vi "Remove Unprintable Chars.vi"(1 "input":string caption="Eingang") -> (0 "output":string caption="Ausgang")   [LabVIEW 2009]
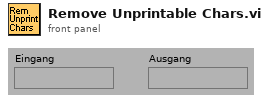
[diagram p1: front panel]
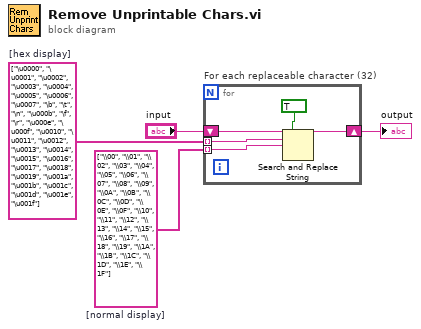
[diagram p0: block diagram]
diagram:
  w2 = string[] ["\u0000", "\u0001", "\u0002", "\u0003", "\u0004", "\u0005", "\u0006", "\u0007", "\b", "\t", "\n", "\u000b", "\f", "\r", "\u000e", "\u000f", "\u0010", "\u0011", "\u0012", "\u0013", "\u0014", "\u0015", "\u0016", "\u0017", "\u0018", "\u0019", "\u001a", "\u001b", "\u001c", "\u001d", "\u001e", "\u001f"]  # [hex display]
  w4 = string[] ["\\00", "\\01", "\\02", "\\03", "\\04", "\\05", "\\06", "\\07", "\\08", "\\09", "\\0A", "\\0B", "\\0C", "\\0D", "\\0E", "\\0F", "\\10", "\\11", "\\12", "\\13", "\\14", "\\15", "\\16", "\\17", "\\18", "\\19", "\\1A", "\\1B", "\\1C", "\\1D", "\\1E", "\\1F"]  # [normal display]
  n1 = for "For each replaceable character (32)" {
    shift-right: [w8] -> w3
    shift-left: "input" -> [w9]
    tunnel: w4 -> [w7] mode=indexing
    tunnel: w2 -> [w6] mode=indexing
    n2 = Search and Replace String(replace all?=TRUE ("replace all? (F)"), input string=w9, search string=w6, replace string=w7) -> (result string=w8:string)  [unwired: 4 in, 3 out]
  }
  "output" <- w3
